vi "Configure NPLC Caching.vi"(8 "error in (no error)":errorcluster, 9 "Cache Operation (0: Reset)":u16(ring) items=["Reset", "Update"], 10 "Enable NPLC Caching (T:Enable)":bool=TRUE, 11 "VISA resource name":refnum<visa-resource-name>) -> (0 "error out":errorcluster, 3 "VISA resource name out":refnum<visa-resource-name>)   [LabVIEW 2012, in "Keithley 24XX.lvlib"]
doc: "Enables the NPLC Cache and resets or updates it. This can be useful to speed up sampling of a measurement at the cost of accuracy."
uses:
  <instrlib>/Keithley 24XX/Keithley 24XX.lvlib
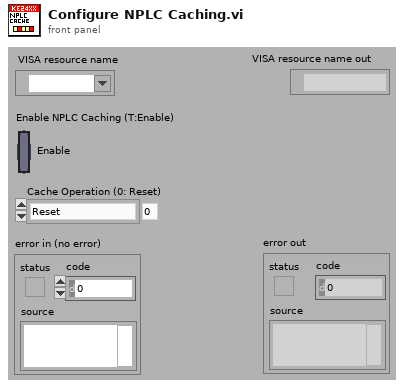
[diagram p1: front panel]
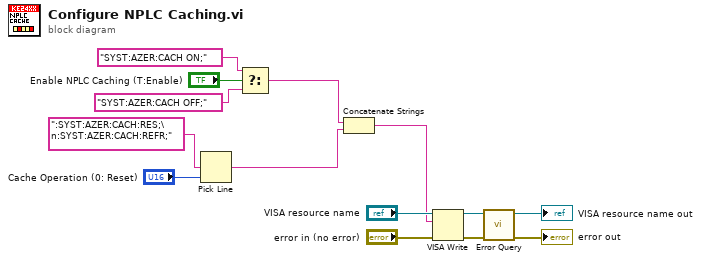
[diagram p0: block diagram]
diagram:
  n1 = Pick Line(multi-line string=":SYST:AZER:CACH:RES;\n:SYST:AZER:CACH:REFR;", line index="Cache Operation (0: Reset)") -> (output string=w3:string)  [unwired: 1 in]
  n2 = Select(t="SYST:AZER:CACH ON;", s="Enable NPLC Caching (T:Enable)", f="SYST:AZER:CACH OFF;") -> (s? t:f=w2:string)
  n3 = Concatenate Strings(w2, w3) -> (w1:string)
  n4 = VISA Write(VISA resource name="VISA resource name", write buffer=w1, error in (no error)="error in (no error)") -> (VISA resource name out=w10:refnum<visa-resource-name>, error out=w9:errorcluster)  [unwired: 1 out]
  n5 = call <instrlib>:"Error Query.vi"("error in (no error)"=w9, "VISA resource name"=w10) -> ("error out"=→"error out":errorcluster, "VISA resource name out"=→"VISA resource name out":refnum<visa-resource-name>)  [unwired: 6 in, 2 out]
